vi "M_D_Archivos.vi"() -> ()   [LabVIEW 2021]
panel:
  out "text":string[](array[string])
  in  "file path (use dialog)":path
  # "Mendoza Meza Manuel Everardo"
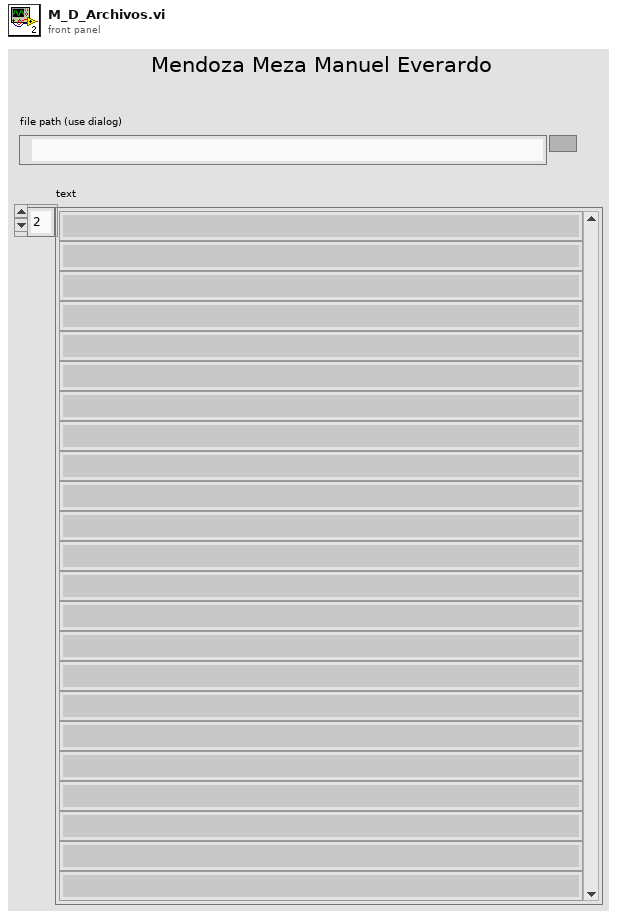
[diagram p1: front panel]
types:
  T1 = enum16{"open", "replace", "create", "open or create", "replace or create", "replace or create with confirmation"}
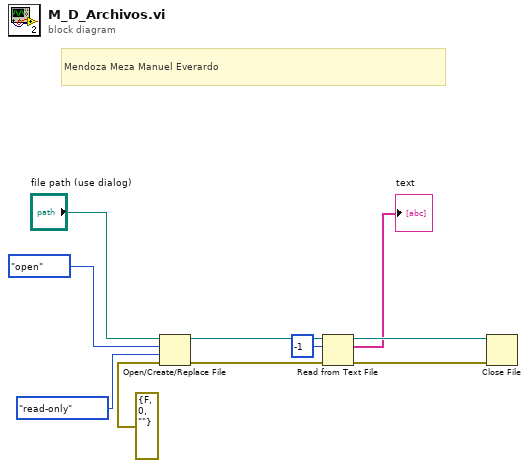
[diagram p0: block diagram]
diagram:
  # "Mendoza Meza Manuel Everardo"
  n1 = Open/Create/Replace File(file path (use dialog)="file path (use dialog)", error in=errorcluster {"status"=FALSE, "code"=0, "source"=""}, operation (0:open)=T1."open", access (0:read/write)=enum16{"read/write", "read-only", "write-only"}."read-only") -> (refnum out=w10:refnum<file>, error out=w8:errorcluster)  [unwired: 2 in, 1 out]
  n2 = Read from Text File(file (use dialog)=w10, count=-1, error in=w8) -> (refnum out=w9:refnum<file>, text=→"text":string[], error out=w7:errorcluster)  [unwired: 1 in, 1 out]
  n3 = Close File(refnum=w9, error in=w7) -> ()  [unwired: 2 out]
